vi "Add Obstacles.vi"(1 "Map":bool[][](array[boolean]), 2 "Obstacles":dbl[](array[numeric])) -> (0 "Map With Obstacles":bool[][](array[boolean]))   [LabVIEW 2015]
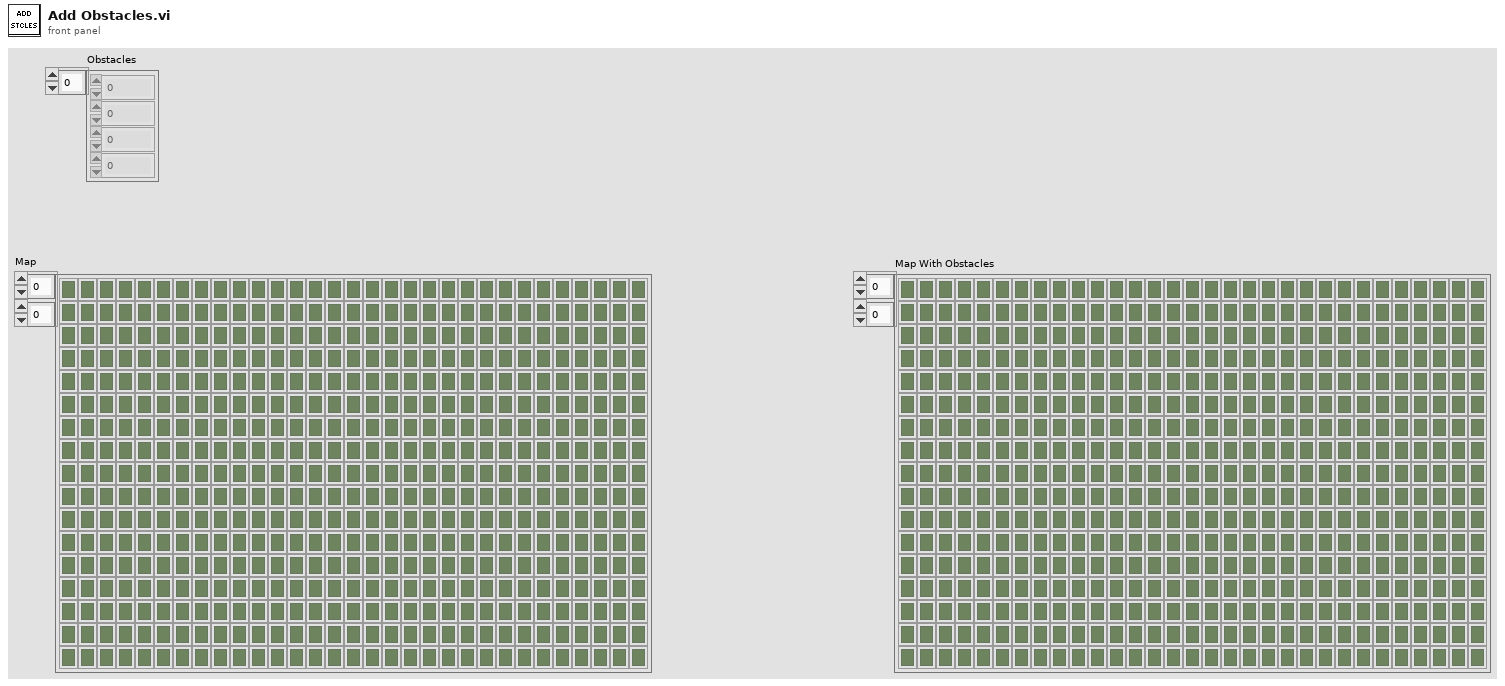
[diagram p1: front panel]
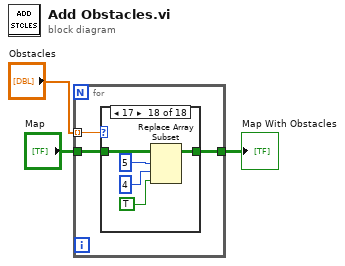
[diagram p0: block diagram]
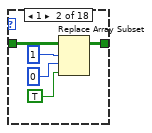
[diagram p3: hidden frame]
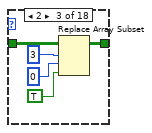
[diagram p4: hidden frame]
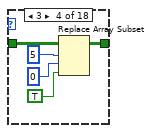
[diagram p5: hidden frame]
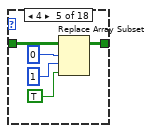
[diagram p6: hidden frame]
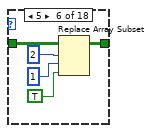
[diagram p7: hidden frame]
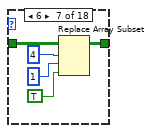
[diagram p8: hidden frame]
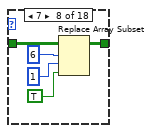
[diagram p9: hidden frame]
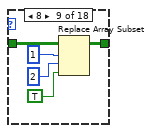
[diagram p10: hidden frame]
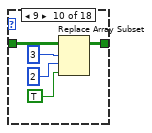
[diagram p11: hidden frame]
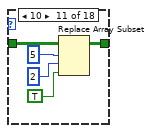
[diagram p12: hidden frame]
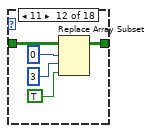
[diagram p13: hidden frame]
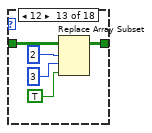
[diagram p14: hidden frame]
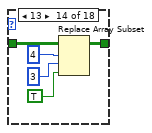
[diagram p15: hidden frame]
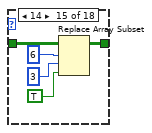
[diagram p16: hidden frame]
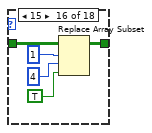
[diagram p17: hidden frame]
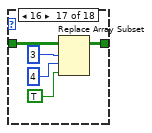
[diagram p18: hidden frame]
diagram:
  n1 = for {
    tunnel: "Obstacles" -> [w6] mode=indexing
    tunnel: "Map" -> [w5]
    tunnel: [w4] -> w1
    n2 = case shown="17" w6 {
      tunnel: w5 -> [w7 w12 w17 w22 w27 w32 w37 w42 w47 w52 w57 w62 w67 w72 w77 w82 w87 w92]
      tunnel: [w7 w8 w13 w18 w23 w28 w33 w38 w43 w48 w53 w58 w63 w68 w73 w78 w83 w88] -> w4
      frame 0, Default {
      }
      frame 1 {
        n3 = Replace Array Subset(array=w12, new element=TRUE ("new element/subarray"), index (row)=1, index (col)=0 ("disabled index (col)")) -> (w8:bool[][])
      }
      frame 2 {
        n4 = Replace Array Subset(array=w17, new element=TRUE ("new element/subarray"), index (row)=3, index (col)=0 ("disabled index (col)")) -> (w13:bool[][])
      }
      frame 3 {
        n5 = Replace Array Subset(array=w22, new element=TRUE ("new element/subarray"), index (row)=5, index (col)=0 ("disabled index (col)")) -> (w18:bool[][])
      }
      frame 4 {
        n6 = Replace Array Subset(array=w27, new element=TRUE ("new element/subarray"), index (row)=0, index (col)=1 ("disabled index (col)")) -> (w23:bool[][])
      }
      frame 5 {
        n7 = Replace Array Subset(array=w32, new element=TRUE ("new element/subarray"), index (row)=2, index (col)=1 ("disabled index (col)")) -> (w28:bool[][])
      }
      frame 6 {
        n8 = Replace Array Subset(array=w37, new element=TRUE ("new element/subarray"), index (row)=4, index (col)=1 ("disabled index (col)")) -> (w33:bool[][])
      }
      frame 7 {
        n9 = Replace Array Subset(array=w42, new element=TRUE ("new element/subarray"), index (row)=6, index (col)=1 ("disabled index (col)")) -> (w38:bool[][])
      }
      frame 8 {
        n10 = Replace Array Subset(array=w47, new element=TRUE ("new element/subarray"), index (row)=1, index (col)=2 ("disabled index (col)")) -> (w43:bool[][])
      }
      frame 9 {
        n11 = Replace Array Subset(array=w52, new element=TRUE ("new element/subarray"), index (row)=3, index (col)=2 ("disabled index (col)")) -> (w48:bool[][])
      }
      frame 10 {
        n12 = Replace Array Subset(array=w57, new element=TRUE ("new element/subarray"), index (row)=5, index (col)=2 ("disabled index (col)")) -> (w53:bool[][])
      }
      frame 11 {
        n13 = Replace Array Subset(array=w62, new element=TRUE ("new element/subarray"), index (row)=0, index (col)=3 ("disabled index (col)")) -> (w58:bool[][])
      }
      frame 12 {
        n14 = Replace Array Subset(array=w67, new element=TRUE ("new element/subarray"), index (row)=2, index (col)=3 ("disabled index (col)")) -> (w63:bool[][])
      }
      frame 13 {
        n15 = Replace Array Subset(array=w72, new element=TRUE ("new element/subarray"), index (row)=4, index (col)=3 ("disabled index (col)")) -> (w68:bool[][])
      }
      frame 14 {
        n16 = Replace Array Subset(array=w77, new element=TRUE ("new element/subarray"), index (row)=6, index (col)=3 ("disabled index (col)")) -> (w73:bool[][])
      }
      frame 15 {
        n17 = Replace Array Subset(array=w82, new element=TRUE ("new element/subarray"), index (row)=1, index (col)=4 ("disabled index (col)")) -> (w78:bool[][])
      }
      frame 16 {
        n18 = Replace Array Subset(array=w87, new element=TRUE ("new element/subarray"), index (row)=3, index (col)=4 ("disabled index (col)")) -> (w83:bool[][])
      }
      frame 17 {
        n19 = Replace Array Subset(array=w92, new element=TRUE ("new element/subarray"), index (row)=5, index (col)=4 ("disabled index (col)")) -> (w88:bool[][])
      }
    }
  }
  "Map With Obstacles" <- w1
